vi "CRYUpdate Tree Indent.vi"(0 "sOption":string, 5 "Open States In":bool[](array[boolean]), 7 "Source Index":i32, 9 "SourceCount":i32, 11 "Target Index":i32) -> (4 "Open States Out":bool[](array[boolean]))   [LabVIEW 2013]
panel:
  out "Test Array Out":string[](array[string])
  in  "Test Array In":string[](array[string])
  in  "Move Up":bool
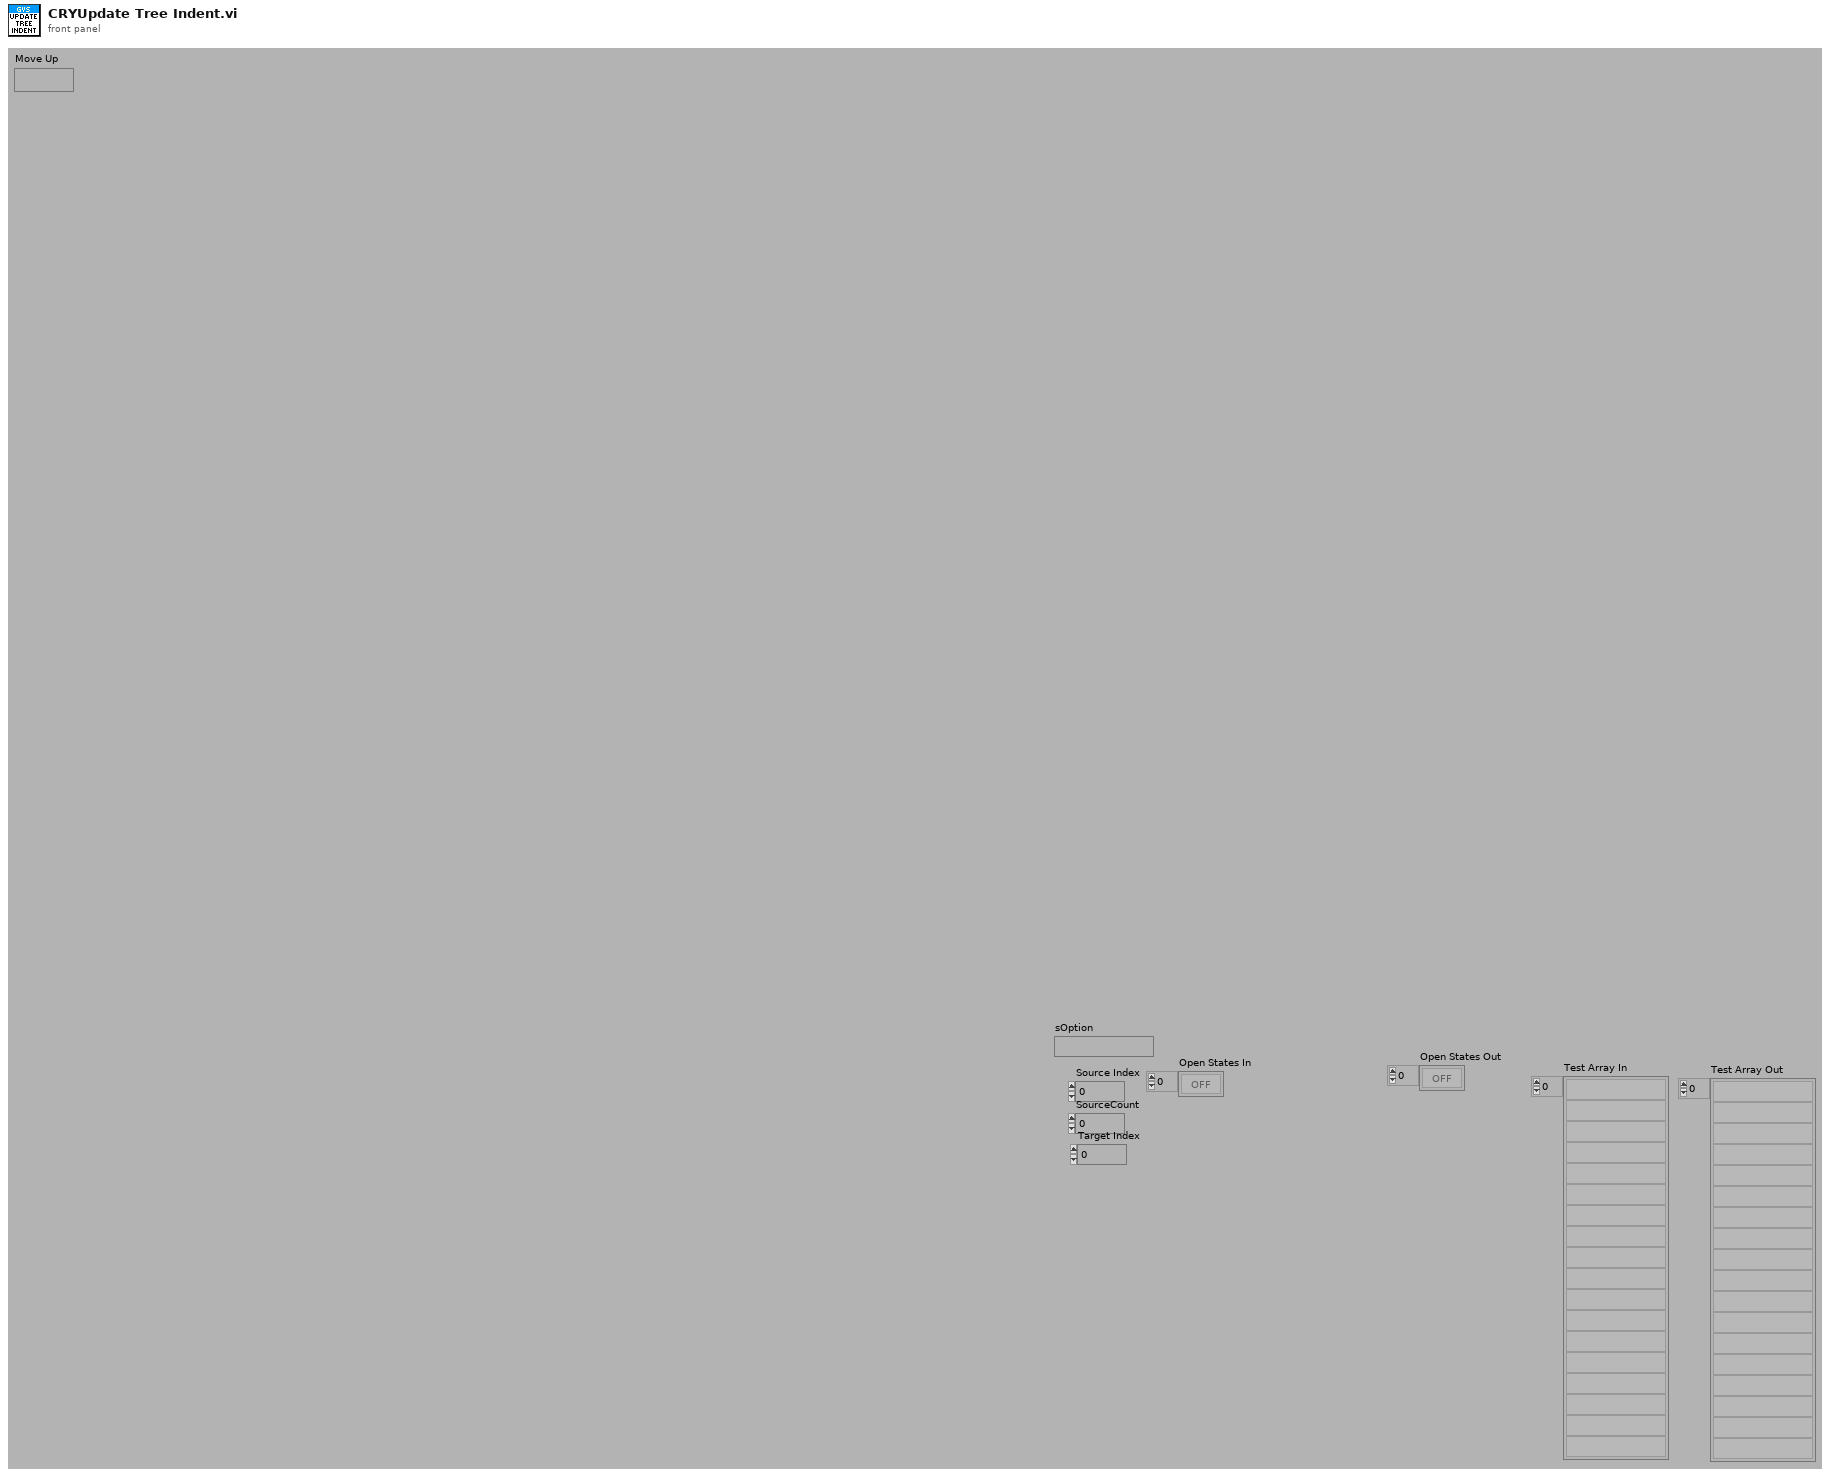
[diagram p1: front panel]
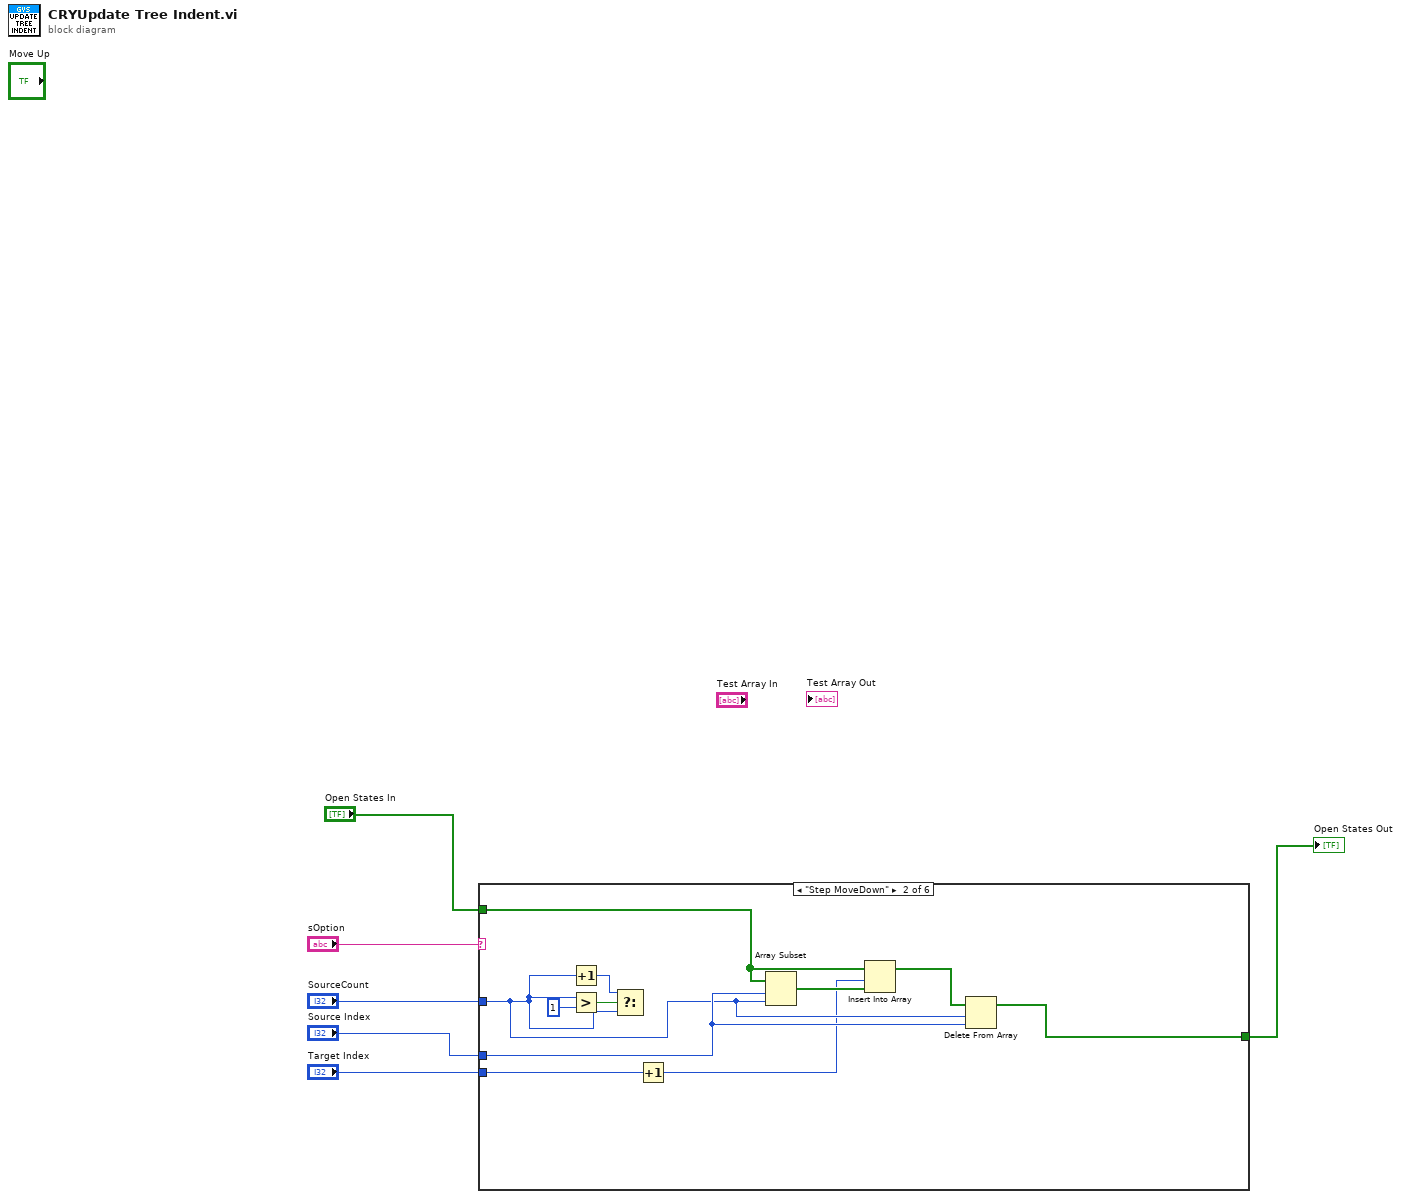
[diagram p0: block diagram]
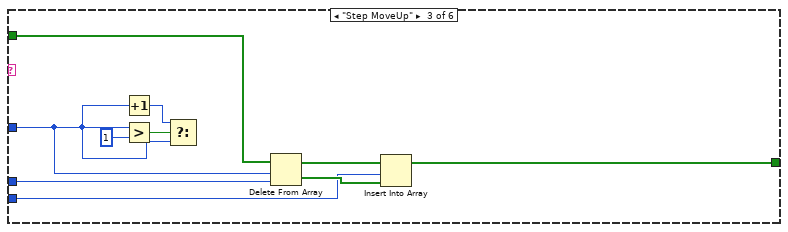
[diagram p3: hidden frame]
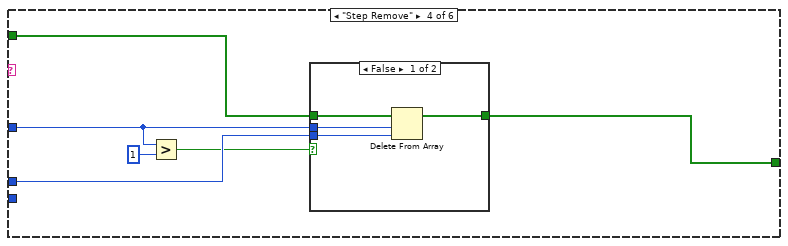
[diagram p4: hidden frame]
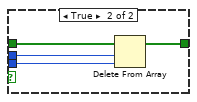
[diagram p5: hidden frame]
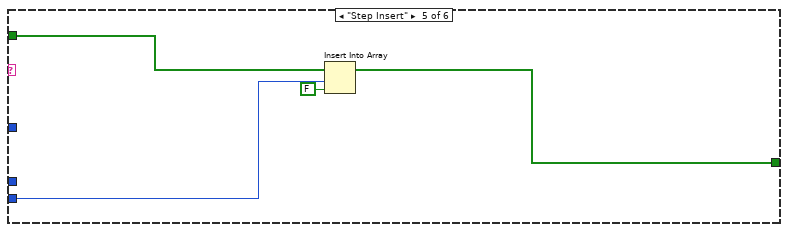
[diagram p6: hidden frame]
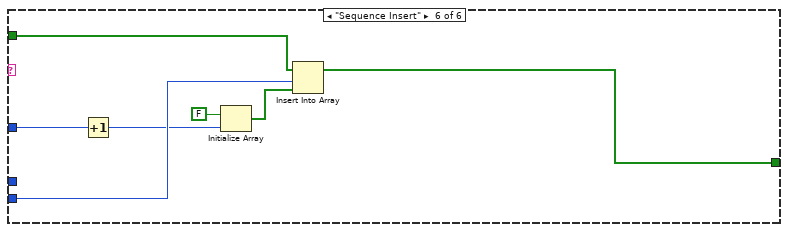
[diagram p7: hidden frame]
diagram:
  n1 = case shown="\"Step MoveDown\"" "sOption" {
    tunnel: "SourceCount" -> [_ w9 w19 w31 _ w49]
    tunnel: "Source Index" -> [_ w16 w25 w34 _ _]
    tunnel: "Open States In" -> [w7 w14 w26 w32 w46 w53]
    tunnel: "Target Index" -> [_ w15 w27 _ w45 w51]
    tunnel: [w7 w13 w24 w33 w43 w52] -> w1
    frame Default {
    }
    frame "Step MoveDown" {
      n2 = Increment(x=w9) -> (x+1=w10:i32)
      n3 = Greater?(x=w9, y=1) -> (0:w11:bool)
      n4 = Select(t=w10, s=w11, f=w9) -> ()  [unwired: 1 out]
      n5 = Increment(x=w15) -> (x+1=w8:i32)
      n6 = Array Subset(array=w14, index=w16, length=w9) -> (w18:bool[])
      n7 = Insert Into Array(array=w14, index=w8, new element=w18) -> (w17:bool[])
      n8 = Delete From Array(array=w17, length=w9, index=w16) -> (array with subset deleted=w13:bool[])  [unwired: 1 out]
    }
    frame "Step MoveUp" {
      n9 = Increment(x=w19) -> (x+1=w20:i32)
      n10 = Greater?(x=w19, y=1) -> (0:w21:bool)
      n11 = Select(t=w20, s=w21, f=w19) -> ()  [unwired: 1 out]
      n12 = Delete From Array(array=w26, length=w19, index=w25) -> (deleted portion=w28:bool[], array with subset deleted=w23:bool[])
      n13 = Insert Into Array(array=w23, index=w27, new element=w28) -> (w24:bool[])
    }
    frame "Step Remove" {
      n14 = Greater?(x=w31, y=1) -> (0:w29:bool)
      n15 = case shown="False" w29 {
        tunnel: w34 -> [w35 w42]
        tunnel: [w37 w41] -> w33
        tunnel: w32 -> [w38 w40]
        tunnel: w31 -> [w36 w39]
        frame False {
          n16 = Delete From Array(array=w38, length=w36, index=w35) -> (array with subset deleted=w37:bool[])  [unwired: 1 out]
        }
        frame True {
          n17 = Delete From Array(array=w40, length=w39, index=w42) -> (array with subset deleted=w41:bool[])  [unwired: 1 out]
        }
      }
    }
    frame "Step Insert" {
      n18 = Insert Into Array(array=w46, index=w45, new element=FALSE ("new element/subarray")) -> (w43:bool[])
    }
    frame "Sequence Insert" {
      n19 = Increment(x=w49) -> (x+1=w48:i32)
      n20 = Initialize Array(FALSE ("new element/subarray"), w48) -> (w47:bool[])
      n21 = Insert Into Array(array=w53, index=w51, new element=w47) -> (w52:bool[])
    }
  }
  "Open States Out" <- w1
